vi "0506_Identificador_de_objetos.vi"() -> ()   [LabVIEW 2017]
uses:
  <vilib>/userdefined/High Color/IMAQdx.ctl
  <vilib>/vision/driver/IMAQdx.llb/IMAQdx Acquisition Mode.ctl
  <vilib>/vision/driver/IMAQdx.llb/IMAQdx Buffer Number Mode.ctl
  <vilib>/vision/driver/NI_Vision_Acquisition_Software.lvlib
  <vilib>/vision/NI_Vision_Development_Module.lvlib
panel:
  out "Boolean":bool
  in  "Settings":T1={"Objects"=0, "Threshold"=128, "Reject Border"=FALSE, "Fill Holes"=FALSE, "Min Object Size"=FALSE, "Min Size"=3, "Max Object Size"=FALSE, "Max Size"=100, "Show Search Area"=FALSE, "Show Center"=TRUE, "Show Bounding Box"=TRUE} {"Objects" items=["Bright Objects", "Dark Objects"]; "Threshold" min=1 max=999999999 step=1; "Max Size" min=1 max=999999999 step=1; "Min Size" min=1 max=999999999 step=1}
  in  "Color Mode":u16(ring) items=["RGB", "HSL", "HSV", "HSI"]
  in  "Red or Hue Range":cluster{"Lower value":sgl, "Upper value":sgl}={"Lower value"=0.0, "Upper value"=255.0} {"Upper value" scale=0.0..255.0; "Lower value" scale=0.0..255.0}
  in  "Green or Sat Range":cluster{"Lower value":sgl, "Upper value":sgl}={"Lower value"=0.0, "Upper value"=255.0} {"Upper value" scale=0.0..255.0; "Lower value" scale=0.0..255.0}
  in  "Blue or Luma or Val or Inten Range":cluster{"Lower value":sgl, "Upper value":sgl}={"Lower value"=0.0, "Upper value"=200.09125} {"Upper value" scale=0.0..255.0; "Lower value" scale=0.0..255.0}
  out "Objects":T2(array[cluster]) {"Aspect Ratio" format="%.2f"; "Orientation" format="%.2f"; "Area" format="%.2f"; "Object Center"."Y" format="%.2f"; "Object Center"."X" format="%.2f"}
  out "Imagem Processada":T3(plugin-control)
  out "Imagem Original":T3(plugin-control)
  in  "Stop Button":bool
  out "dt":dbl
  in  "Câmera":T4="cam1"
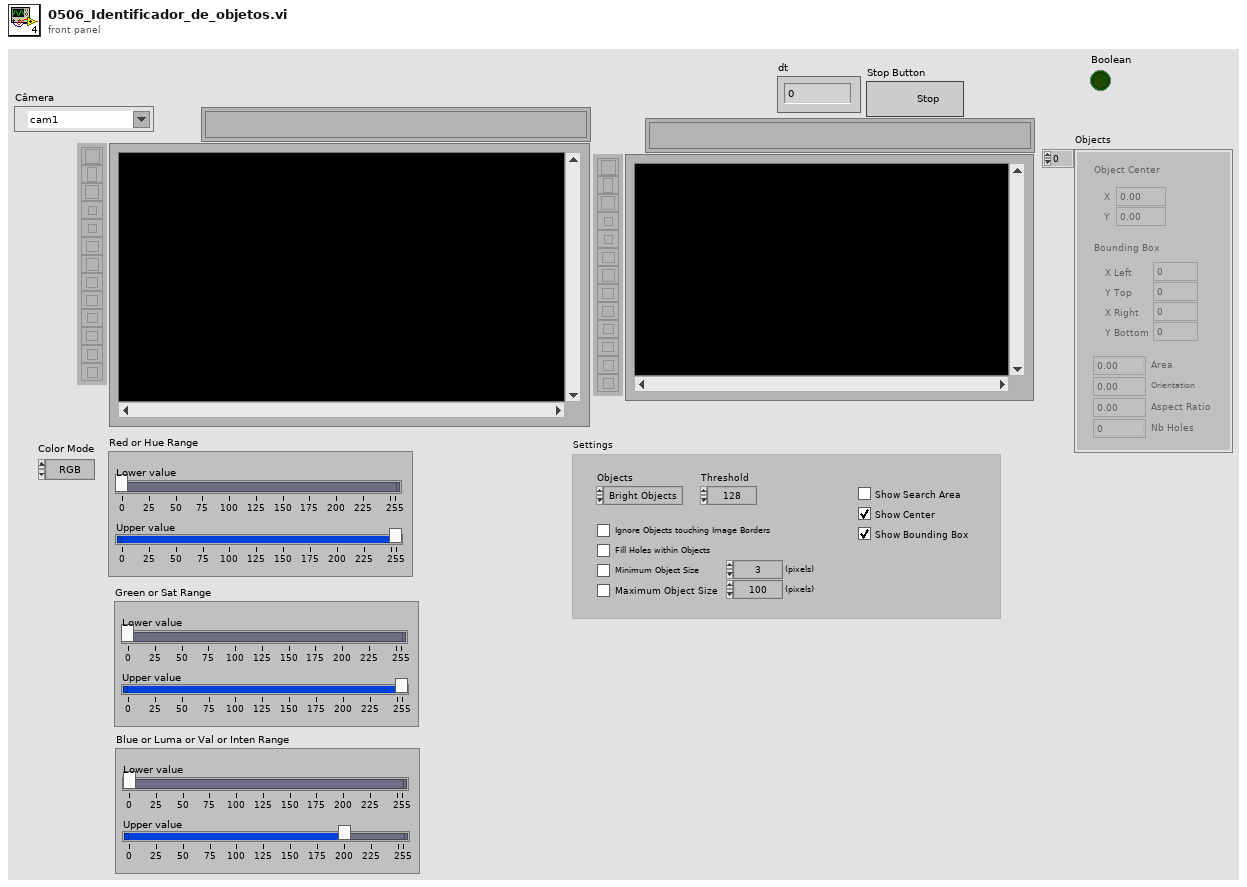
[diagram p1: front panel]
types:
  T1 = cluster{"Objects":u16, "Threshold":i32, "Reject Border":bool, "Fill Holes":bool, "Min Object Size":bool, "Min Size":i32, "Max Object Size":bool, "Max Size":i32, "Show Search Area":bool, "Show Center":bool, "Show Bounding Box":bool}
  T2 = cluster{"Object Center":cluster{"X":sgl, "Y":sgl}, "Bounding Box":cluster{"X Left":i32, "Y Top":i32, "X Right":i32, "Y Bottom":i32}, "Area":sgl, "Orientation":sgl, "Aspect Ratio":sgl, "Nb Holes":i32}[]
  T3 = typedef "IMAQ Image.ctl" = refnum<image>
  T4 = typedef "IMAQdx.ctl" = refnum<k21>
  T5 = typedef "Image Type" = u32
  T6 = typedef "NI_Vision_Acquisition_Software.lvlib/IMAQdx Acquisition Mode.ctl" = enum32{"One Shot", "Continuous"}
  T7 = typedef "NI_Vision_Acquisition_Software.lvlib/IMAQdx Buffer Number Mode.ctl" = enum32{"Next", "Last", "Buffer Number", "Every", "Last New"}
  T8 = cluster{"Global Rectangle":i32[], "Contours":cluster{"Contour Type":u32, "ROI Type":u32, "Points":i32[]}[]}
  T9 = typedef "IMAQ Rectangle" = cluster{"Left":i32, "Top":i32, "Right":i32, "Bottom":i32, "Rotation":dbl}
  T10 = cluster{"Object Center":cluster{"X":sgl, "Y":sgl}, "Bounding Box":cluster{"X Left":i32, "Y Top":i32, "X Right":i32, "Y Bottom":i32}, "Area":sgl, "Orientation":sgl, "Aspect Ratio":sgl, "Nb Holes":i32}
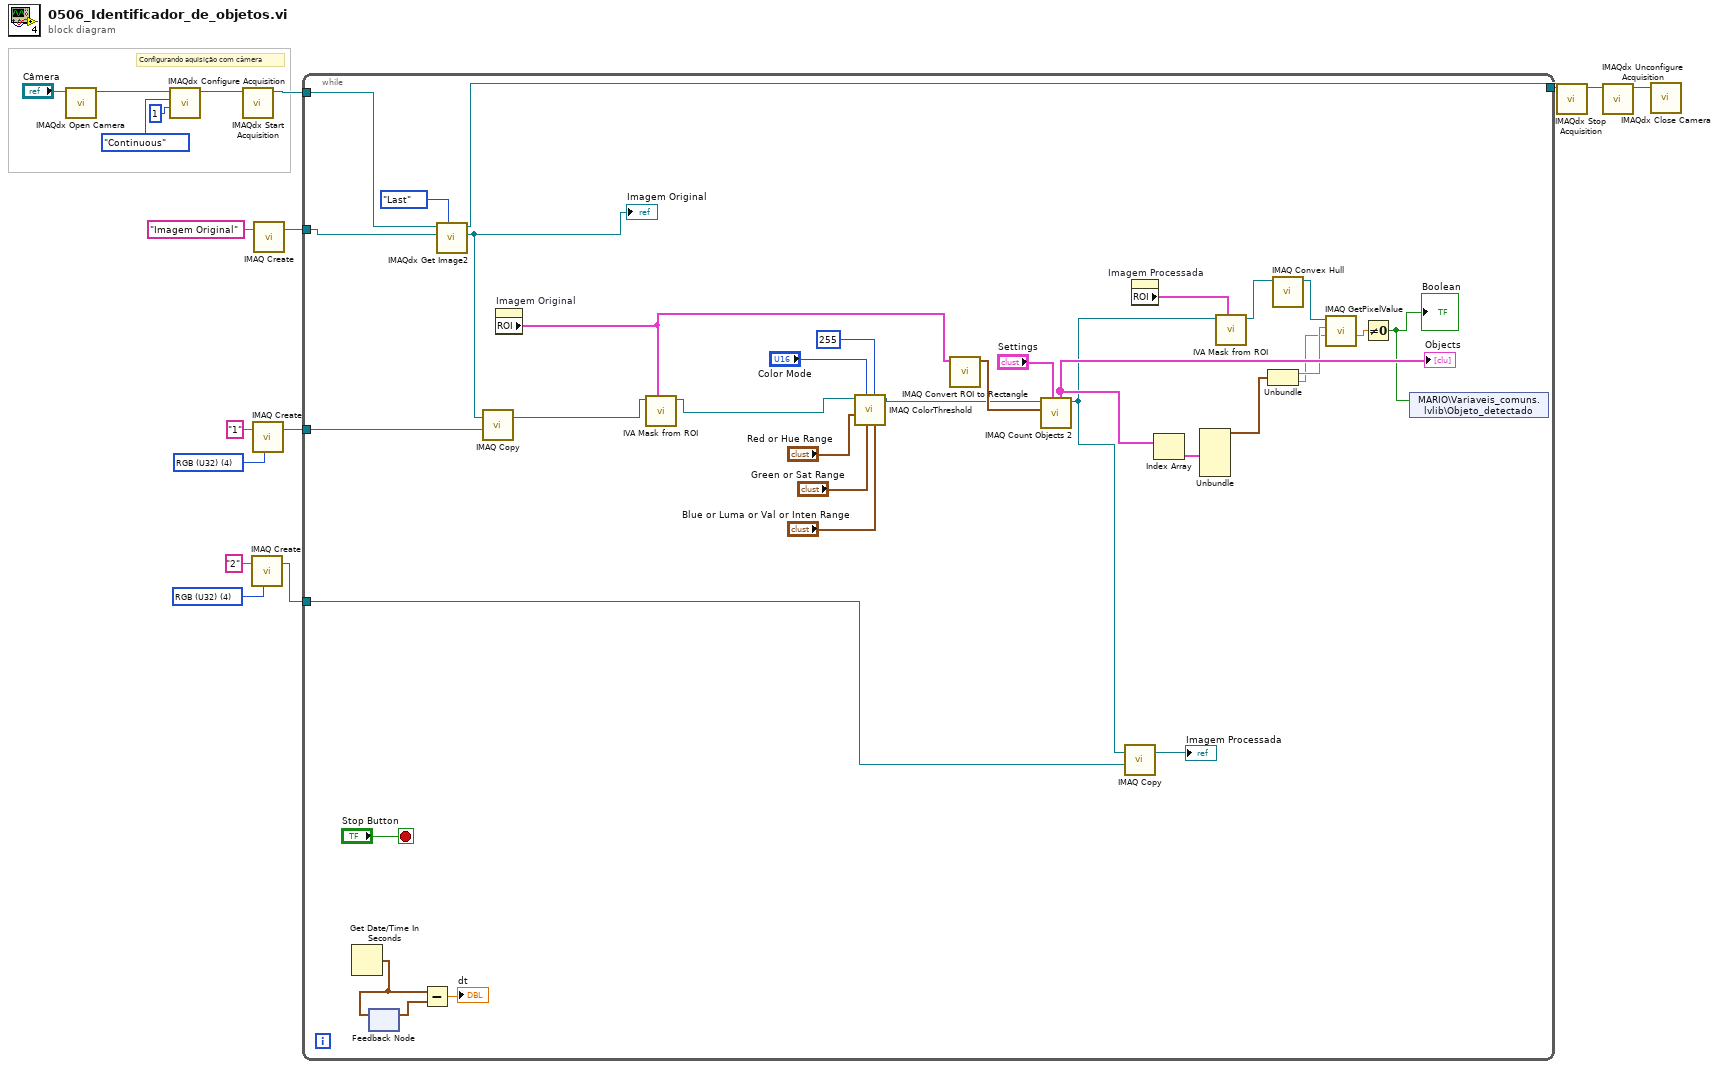
[diagram p0: block diagram]
diagram:
  w6 = T5 4 items=["Grayscale (U8)", "Grayscale (I16)", "Grayscale (SGL)", "Complex (CSG)", "RGB (U32)", "HSL (U32)", "RGB (U64)", "Grayscale (U16)"] ("Image Type")
  w8 = T5 4 items=["Grayscale (U8)", "Grayscale (I16)", "Grayscale (SGL)", "Complex (CSG)", "RGB (U32)", "HSL (U32)", "RGB (U64)", "Grayscale (U16)"] ("Image Type")
  # "Configurando aquisição com câmera"
  n1 = call <vilib>:"IMAQdx Open Camera.vi"("Session In"="Câmera") -> ("Session Out"=w17:T4)  [unwired: 9 in, 1 out]
  n2 = call <vilib>:"IMAQdx Configure Acquisition.vi"("Number of Buffers"=u32 1, "Continuous?"=IMAQdx_Acquisition_Mode."Continuous", "Session In"=w17) -> ("Session Out"=w16:T4)  [unwired: 7 in, 1 out]
  n3 = call <vilib>:"IMAQdx Start Acquisition.vi"("Session In"=w16) -> ("Session Out"=w7:T4)  [unwired: 9 in, 1 out]
  n4 = call "IMAQ Create"("Image Name"="2", "Image Type"=w6) -> ("New Image"=w4:T3)  [unwired: 3 in, 1 out]
  n5 = call "IMAQ Create"("Image Name"="1", "Image Type"=w8) -> ("New Image"=w9:T3)  [unwired: 3 in, 1 out]
  n6 = call "IMAQ Create"("Image Name"="Imagem Original") -> ("New Image"=w13:T3)  [unwired: 4 in, 1 out]
  n7 = while {
    tunnel: w13 -> [w51]
    tunnel: w9 -> [w49]
    tunnel: w7 -> [w48]
    tunnel: [w47] -> w1
    tunnel: w4 -> [w41]
    stop <- "Stop Button" stop-if-true
    n8 = Get Date/Time In Seconds() -> (seconds since 1Jan1904=w44:timestamp)
    n9 = feedback #1() -> (w46:timestamp)  [unwired: 1 in]
    n10 = feedback-in #1(w44) -> ()
    n11 = Subtract(x=w44, y=w46) -> (x-y=→"dt":dbl)
    n12 = call <vilib>:"IMAQdx Get Image2.vi"("Buffer Number Mode (Next)"=IMAQdx_Buffer_Number_Mode."Last", "Image In"=w51, "Session In"=w48) -> ("Image Out"=w23:T3, "Session Out"=w47:T4)  [unwired: 5 in, 2 out]
    "Imagem Original" <- w23
    n13 = call "IMAQ Copy"("Image Dst"=w49, "Image Src"=w23) -> ("Image Dst Out"=w42:T3)  [unwired: 4 in, 1 out]
    n14 = property on="Imagem Original" class="ImageControl"() -> ("ROI"=w32:T8)  [unwired: 2 in, 2 out]
    n15 = call <vilib>:"IVA Mask from ROI.vi"("ROI Descriptor"=w32, "Image Src"=w42) -> ("Image Out"=w34:T3)  [unwired: 3 in, 6 out]
    n16 = call "IMAQ ColorThreshold"("Blue or Luma or Val or Inten Range"="Blue or Luma or Val or Inten Range", "Replace Value"=255, "Green or Sat Range"="Green or Sat Range", "Color Mode"="Color Mode", "Red or Hue Range"="Red or Hue Range", "Image Src"=w34) -> ("Image Dst Out"=w20:T3)  [unwired: 2 in, 3 out]
    n17 = call "IMAQ Convert ROI to Rectangle"("ROI Descriptor"=w32) -> ("Rectangle"=w31:T9)  [unwired: 8 in, 1 out]
    n18 = call "IMAQ Count Objects 2"("Settings"="Settings", "Search Rect (entire image)"=w31, "Image"=w20) -> ("Image Out"=w22:T3, "Objects"=w30:T2)  [unwired: 4 in, 3 out]
    "Objects" <- w30
    n19 = call "IMAQ Copy"("Image Dst"=w41, "Image Src"=w22) -> ("Image Dst Out"=→"Imagem Processada":T3)  [unwired: 4 in, 1 out]
    n20 = property on="Imagem Processada" class="ImageControl"() -> ("ROI"=w25:T8)  [unwired: 2 in, 2 out]
    n21 = Index Array(array=w30) -> (element=w29:T10)  [unwired: 1 in]
    n22 = Unbundle(w29) -> ("Object Center"=w28:cluster{"X":sgl, "Y":sgl})  [unwired: 5 out]
    n23 = call <vilib>:"IVA Mask from ROI.vi"("ROI Descriptor"=w25, "Image Src"=w22) -> ("Image Out"=w19:T3)  [unwired: 3 in, 6 out]
    n24 = Unbundle(w28) -> ("X"=w27:sgl, "Y"=w26:sgl)
    n25 = call "IMAQ Convex Hull"("Image Src"=w19) -> ("Image Dst Out"=w18:T3)  [unwired: 9 in, 1 out]
    n26 = call "IMAQ GetPixelValue"("Image"=w18, "X Coordinate"=w27, "Y Coordinate"=w26) -> ("Pixel Value (Float)"=w24:sgl)  [unwired: 3 in, 4 out]
    n27 = Not Equal To 0?(x=w24) -> (x != 0?=w21:bool)
    "Boolean" <- w21
    n28 = shared-variable "MARIO\\Variaveis_comuns.lvlib\\Objeto_detectado"(w21) -> ()  [unwired: 1 in, 1 out]
  }
  n29 = call <vilib>:"IMAQdx Stop Acquisition.vi"("Session In"=w1) -> ("Session Out"=w3:T4)  [unwired: 9 in, 1 out]
  n30 = call <vilib>:"IMAQdx Unconfigure Acquisition.vi"("Session In"=w3) -> ("Session Out"=w2:T4)  [unwired: 9 in, 1 out]
  n31 = call <vilib>:"IMAQdx Close Camera.vi"("Session In"=w2) -> ()  [unwired: 10 in, 1 out]
